vi "Historical Warnings (SubVI).vi"(7 "Warnings bool array":bool[](array[boolean]), 8 "in":bool, 11 "warnings table in":T1(array[cluster]) {"Time Stamp" format="%<%.3X %x>T"}) -> (3 "Warnings table out":T1(array[cluster]) {"Time Stamp" format="%<%.3X %x>T"})   [LabVIEW 2022 SP3]
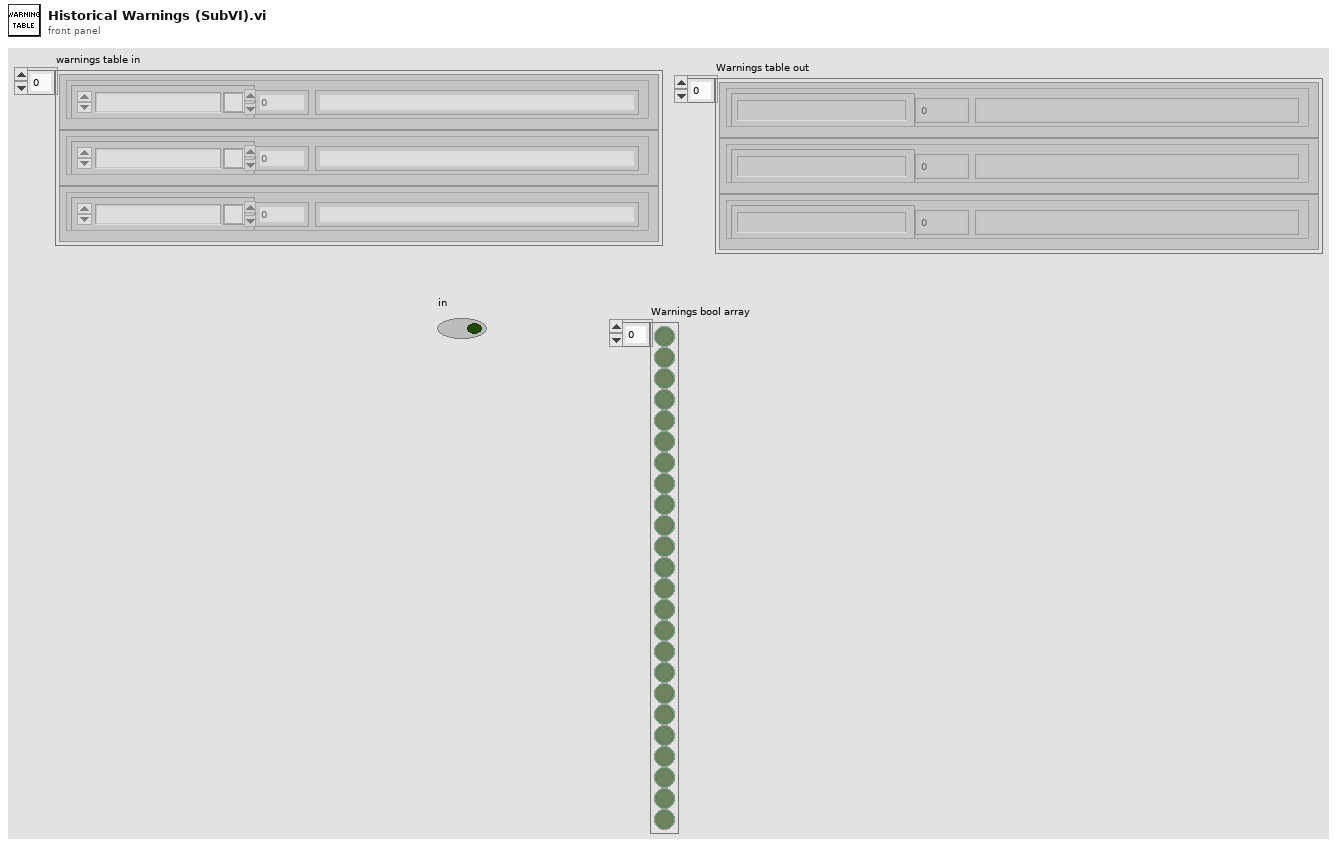
[diagram p1: front panel]
types:
  T1 = cluster{"Time Stamp":timestamp, "Descripcion":string, "Numeric":i32}[]
  T2 = cluster{"Time Stamp":timestamp, "Descripcion":string, "Numeric":i32}
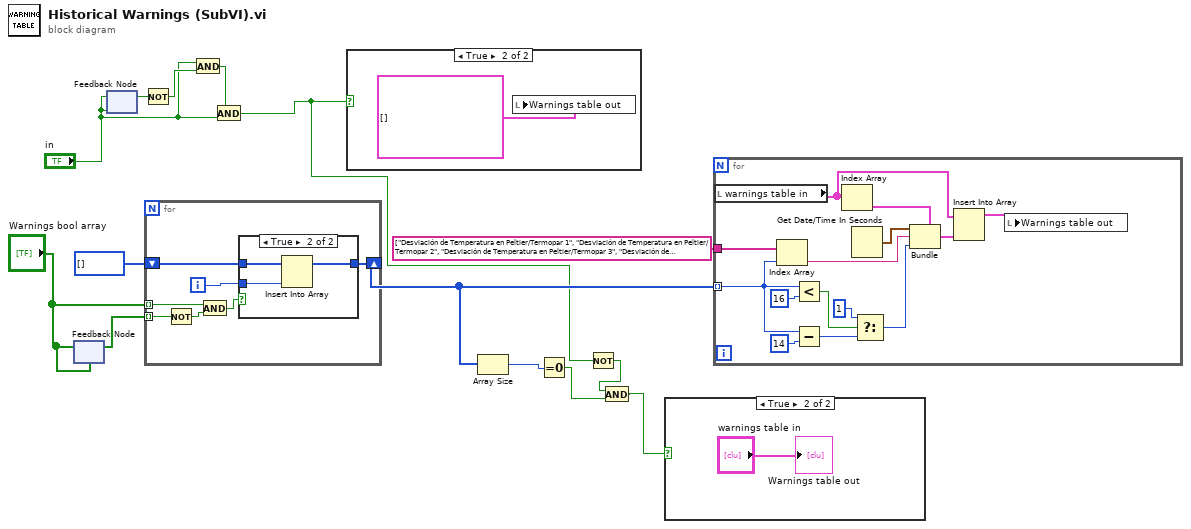
[diagram p0: block diagram]
diagram:
  n1 = feedback #1("Warnings bool array") -> (w11:bool[])
  n2 = feedback-in #1("Warnings bool array") -> ()
  n3 = feedback #2("in") -> (w7:bool)
  n4 = feedback-in #2("in") -> ()
  n5 = Not(x=w7) -> (.not. x?=w8:bool)
  n6 = for {
    tunnel: w11 -> [w21] mode=indexing
    tunnel: "Warnings bool array" -> [w19] mode=indexing
    shift-right: [w15] -> w10
    shift-left: i32[] [] -> [w18]
    i -> [w17]
    n7 = Not(x=w21) -> (.not. x?=w20:bool)
    n8 = And(x=w19, y=w20) -> (x .and. y?=w16:bool)
    n9 = case shown="True" w16 {
      tunnel: w18 -> [w22 w25]
      tunnel: w17 -> [_ w23]
      tunnel: [w22 w24] -> w15
      frame False {
      }
      frame True {
        n10 = Insert Into Array(array=w25, new element=w23) -> (w24:i32[])  [unwired: 1 in]
      }
    }
  }
  n11 = And(x="in", y=w8) -> (x .and. y?=w6:bool)
  n12 = And(x=w6, y="in") -> (x .and. y?=w2:bool)
  n13 = case shown="True" w2 {
    frame False {
    }
    frame True {
      n14 = local write "Warnings table out"(T1 [] ("Warnings table out")) -> ()
    }
  }
  n15 = Array Size(array=w10) -> (size(s)=w9:i32)
  n16 = Equal To 0?(x=w9) -> (x = 0?=w4:bool)
  n17 = Not(x=w2) -> (.not. x?=w3:bool)
  n18 = And(x=w3, y=w4) -> (x .and. y?=w1:bool)
  n19 = case shown="True" w1 {
    frame False {
    }
    frame True {
      "Warnings table out" <- "warnings table in"
    }
  }
  n20 = for {
    tunnel: w10 -> [w30] mode=indexing
    tunnel: string[] ["Desviación de Temperatura en Peltier/Termopar 1", "Desviación de Temperatura en Peltier/Termopar 2", "Desviación de Temperatura en Peltier/Termopar 3", "Desviación de Temperatura en Peltier/Termopar 4", "Desviación de Temperatura en Peltier/Termopar 5", "Desviación de Temperatura en Peltier/Termopar 6", "Desviación de Temperatura en Peltier/Termopar 7", "Desviación de Temperatura en Peltier/Termopar 8", "Desviación de Temperatura en Peltier/Termopar 9", "Desviación de Temperatura en Peltier/Termopar 10", "Desviación de Temperatura en Peltier/Termopar 11", "Desviación de Temperatura en Peltier/Termopar 12", "Desviación de Temperatura en Peltier/Termopar 13", "Desviación de Temperatura en Peltier/Termopar 14", "Desviación de Temperatura en Peltier/Termopar 15", "Desviación de Temperatura en Peltier/Termopar 16", "Desviación de Temperatura en la CC.", "Disparo del valor LEL (%). AMBIENTE EXPLOSIVO", "Valor anómalo de O2(%)"] -> [w38]
    n21 = local read "warnings table in"() -> (w28:T1)
    n22 = Index Array(array=w38, index=w30) -> (element=w37:string)
    n23 = Less?(x=w30, y=16) -> (x < y?=w35:bool)
    n24 = Subtract(x=w30, y=14) -> (x-y=w32:i32)
    n25 = Index Array(array=w28) -> (element=w40:T2)  [unwired: 1 in]
    n26 = Get Date/Time In Seconds() -> (seconds since 1Jan1904=w39:timestamp)
    n27 = Select(t=1, s=w35, f=w32) -> (s? t:f=w31:i32)
    n28 = Bundle(cluster=w40, "Time Stamp"=w39, "Descripcion"=w37, "Numeric"=w31) -> (w41:T2)
    n29 = Insert Into Array(array=w28, new element=w41) -> (w29:T1)  [unwired: 1 in]
    n30 = local write "Warnings table out"(w29) -> ()
  }
